vi "Pre Launch Init.vi"(11 "Nested in":refnum<class "Model_AMC.lvclass">) -> (0 "error out":errorcluster, 3 "Nested out":refnum<class "Model_AMC.lvclass">)   [LabVIEW 2021, in "Model_AMC.lvclass"]
doc: "(<B>Filename</B>: Actor Framework.lvlib:Actor.lvclass:Pre Launch Init.vi)\n\nDefines behavior that occurs after the Launch Nested Actor method is invoked but before the actor's Actor Core method begins running.\n\nBy default, this method does nothing. A descendant class may override it to define behavior."
uses:
  Model_AMC.lvclass
  DVR.ctl
  <userlib>/John_Lib/Network_Streams_Connection/NetworkConnection.lvclass
  AMC Q.ctl
  <userlib>/John_Lib/AMC_FW/AMC_SelfCustom/Queue.ctl
  <userlib>/John_Lib/AMC_FW/Message Queue.ctl
  <userlib>/John_Lib/AMC_FW/Message.ctl
  <userlib>/John_Lib/AMC_FW/Tools/Keyed Array/KeyedArray.ctl
  Model_AMC.lvclass/Model_AMC.ctl
  <userlib>/John_Lib/AbstractActorTemplate/AbstractActorTemplate/UIActorTop.lvclass
  <userlib>/John_Lib/AMC_FW/Tools/Keyed Array/Tools_KeyedArray.lvlib
  <userlib>/John_Lib/AMC_FW/AMC_FW.lvlib
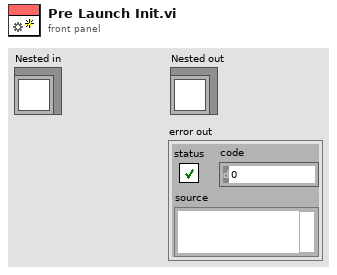
[diagram p1: front panel]
types:
  T1 = typedef "Model_AMC.lvclass/DVR.ctl" = cluster{"JKI_Network_Streams":refnum<class "NetworkConnection.lvclass">, "AMC Q":T2}
  T2 = typedef "Model_AMC.lvclass/AMC Q.ctl" = cluster{"Main":T3, "OPCUA":T3, "NetworkSteam":T3}
  T3 = typedef "AMC_FW.lvlib/Queue.ctl" = cluster{"Q":T4, "Name":string}
  T4 = typedef "AMC_FW.lvlib/Message Queue.ctl" = refnum<queue>
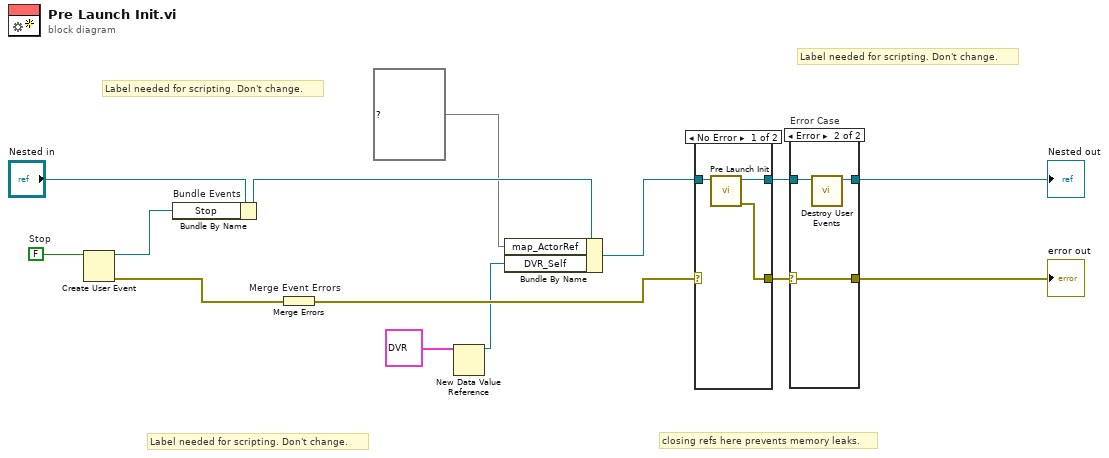
[diagram p0: block diagram]
diagram:
  w13 = FALSE  # Stop
  # "Label needed for scripting. Don't change."
  # "Label needed for scripting. Don't change."
  # "Label needed for scripting. Don't change."
  # "closing refs here prevents memory leaks."
  n1 = Create User Event(user event datatype=w13) -> (user event=w10:refnum<user-event>, error out=w12:errorcluster)  [unwired: 1 in]
  n2 = Bundle By Name "Bundle Events"(cluster="Nested in", "Stop"=w10) -> (w4:refnum<class "Model_AMC.lvclass">)
  n3 = Merge Errors "Merge Event Errors"(w12) -> (w7:errorcluster)
  n4 = New Data Value Reference(data value=T1 {"JKI_Network_Streams"=refnum, "AMC Q"={"Main"={"Q"=refnum, "Name"=""}, "OPCUA"={"Q"=refnum, "Name"=""}, "NetworkSteam"={"Q"=refnum, "Name"=""}}} ("DVR")) -> (data value reference=w1:refnum<data-value>)  [unwired: 1 in, 1 out]
  n5 = Bundle By Name(cluster=w4, "map_ActorRef"=map{string, refnum<vi>} {}, "DVR_Self"=w1) -> (w3:refnum<class "Model_AMC.lvclass">)
  n6 = case shown="No Error" w7 {
    selector: w7 -> [_ w19]
    tunnel: [w17 w18] -> w8
    tunnel: w3 -> [w16 w18]
    tunnel: [w15 w19] -> w6
    frame No Error {
      n7 = call-parent "Pre Launch Init.vi"("Actor in"=w16) -> ("error out"=w15:errorcluster, "Actor out"=w17:refnum<class "Model_AMC.lvclass">)  [unwired: 9 in]
    }
    frame Error {
    }
  }
  n8 = case "Error Case" shown="Error" w6 {
    selector: w6 -> [w20 w24]
    tunnel: w8 -> [w21 w23]
    tunnel: [w21 w22] -> w11
    tunnel: [w20 w24] -> w9
    frame No Error {
    }
    frame Error {
      n9 = call "Destroy User Events.vi"("UI Template in"=w23) -> ("UI Template out"=w22:refnum<class "Model_AMC.lvclass">)  [unwired: 10 in]
    }
  }
  "error out" <- w9
  "Nested out" <- w11
